vi "定时启动 (子VI).vi"   [LabVIEW 2016, in "斯坦道CODMn.lvlib"]
types:
  T1 = enum16{"启动测量", "标样核查", "零点核查", "跨度核查", "空白测试", "平行样测试", "加标回收", "空白校准", "标样校准", "初始化（清洗）", "停止测试", "仪器重启", "校时", "模式设置", "测量间隔设置"}
  T2 = cluster{"测量模式":enum16{"水样测量", "标样核查", "零点核查", "跨度核查", "空白测试", "加标回收", "平行样", "校零", "校标"}}
  T3 = cluster{"控制命令":enum16{"启动测量", "标样核查", "零点核查", "跨度核查", "空白测试", "平行样测试", "加标回收", "空白校准", "标样校准", "初始化（清洗）", "停止测试", "仪器重启", "校时", "模式设置", "测量间隔设置"}, "周期设置类型":enum16{"定点启动", "间隔启动"}, "定时功能启用":bool, "定时间隔":dbl, "24H周期设置":bool[], "零点核查时间":u16, "跨度核查时间":u16, "质控频次":enum16{"关闭", "每天", "星期一", "星期二", "星期三", "星期四", "星期五", "星期六", "星期日"}}
  T4 = enum16{"关闭", "每天", "星期一", "星期二", "星期三", "星期四", "星期五", "星期六", "星期日"}
  T5 = typedef "LVDateTimeRec.ctl" = cluster{"秒数的小数部分":dbl, "秒":i32, "分":i32, "时":i32, "日":i32, "月":i32, "年":i32, "天数（周）":i32, "天数（年）":i32, "DST":i32}
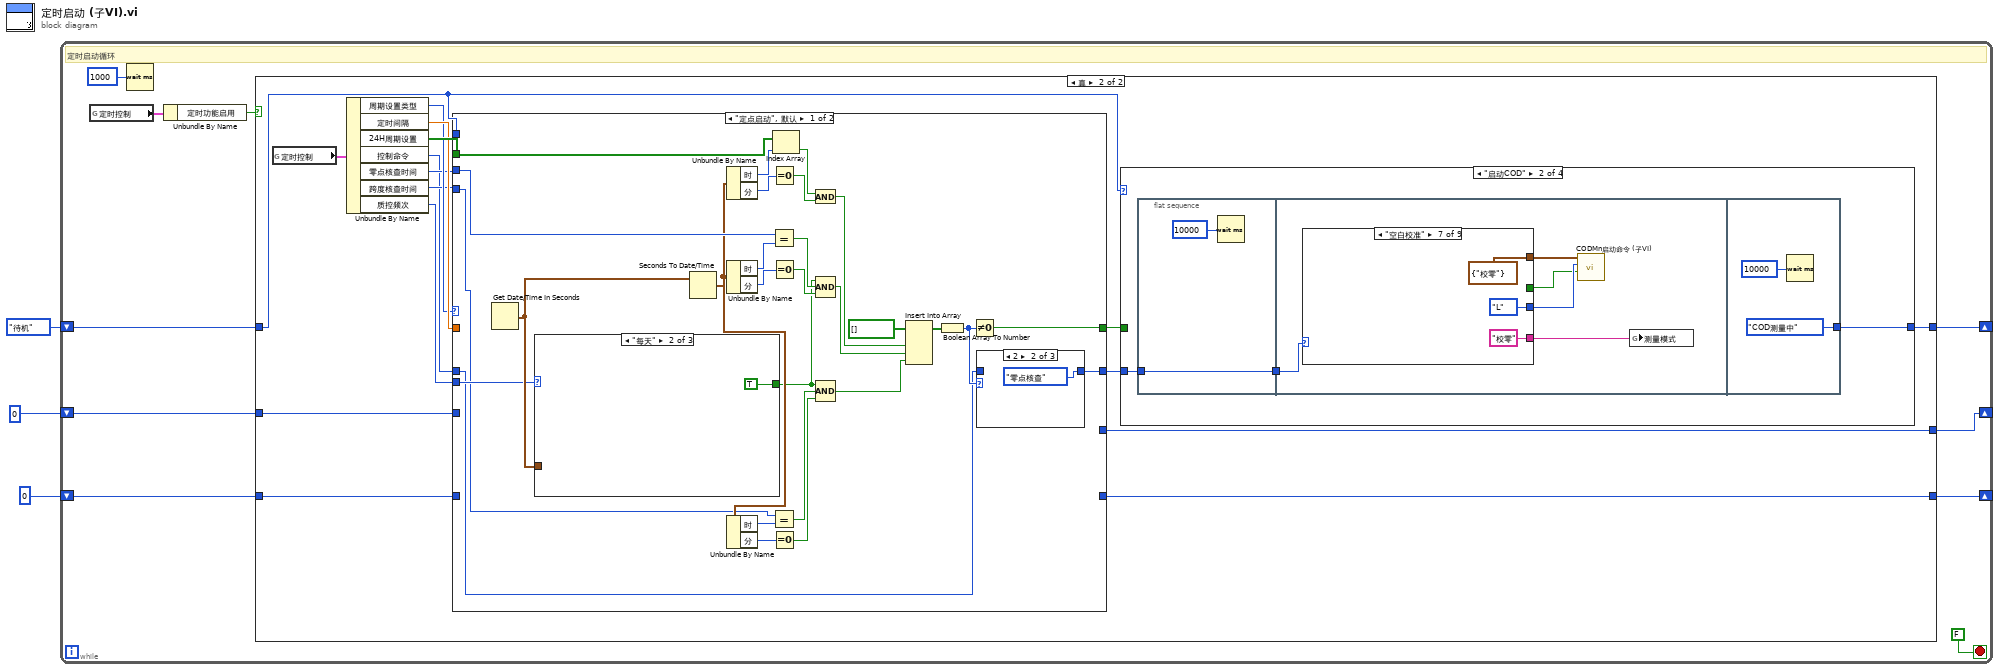
[diagram p0: block diagram]
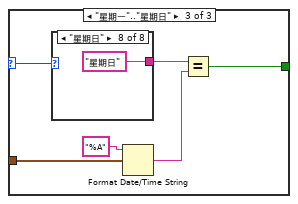
[diagram p4: hidden frame]
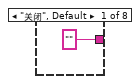
[diagram p5: hidden frame]
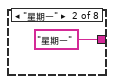
[diagram p6: hidden frame]
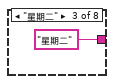
[diagram p7: hidden frame]
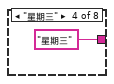
[diagram p8: hidden frame]
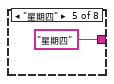
[diagram p9: hidden frame]
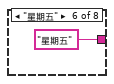
[diagram p10: hidden frame]
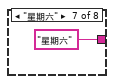
[diagram p11: hidden frame]
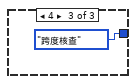
[diagram p13: hidden frame]
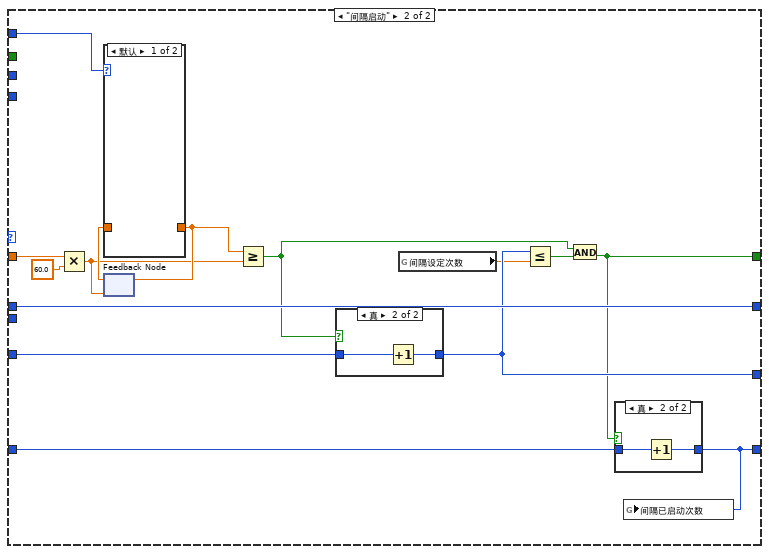
[diagram p14: hidden frame]
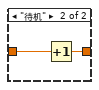
[diagram p17: hidden frame]
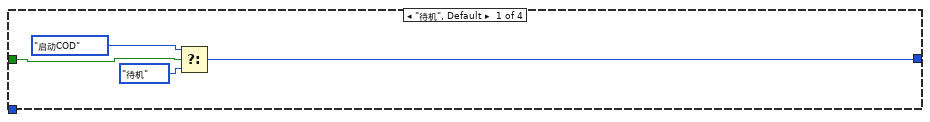
[diagram p18: hidden frame]
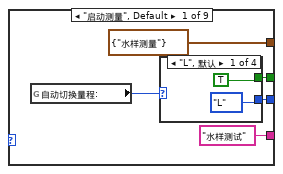
[diagram p19: hidden frame]
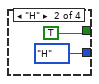
[diagram p20: hidden frame]
diagram:
  n1 = while {
    shift-right: [w12] -> _
    shift-left: enum16{"待机", "启动COD", "COD测量中", "延时"}."待机" -> [w11]
    shift-right: [w6] -> _
    shift-left: 0 -> [w7]
    shift-right: [w4] -> _
    shift-left: 0 -> [w5]
    stop <- FALSE stop-if-true
    # "定时启动循环"
    n2 = global read "CODMn断电保存全局变量.vi" "定时控制"() -> (w10:T3)
    n3 = Wait (ms)(milliseconds to wait=u32 1000 ("等待时间（毫秒）")) -> ()  [unwired: 1 out]
    n4 = Unbundle By Name(w10) -> ("定时功能启用"=w9:bool)
    n5 = case shown="真" w9 {
      tunnel: [w14 w30] -> w12
      tunnel: w11 -> [w14 w29]
      tunnel: w7 -> [_ w18]
      tunnel: [_ w17] -> w6
      tunnel: w5 -> [_ w16]
      tunnel: [_ w15] -> w4
      frame False {
      }
      frame True {
        n6 = global read "CODMn断电保存全局变量.vi" "定时控制"() -> (w23:T3)
        n7 = Unbundle By Name(w23) -> ("周期设置类型"=w24:enum16{"定点启动", "间隔启动"}, "定时间隔"=w25:dbl, "24H周期设置"=w26:bool[], "控制命令"=w19:T1, "零点核查时间"=w22:u16, "跨度核查时间"=w20:u16, "质控频次"=w21:T4)
        n8 = case shown="\"定点启动\", 默认" w24 {
          tunnel: w25 -> [_ w88]
          tunnel: w26 -> [w58 _]
          tunnel: w29 -> [_ w91]
          tunnel: [w34 w80] -> w28
          tunnel: w22 -> [w57 _]
          tunnel: w21 -> [w35 _]
          tunnel: w20 -> [w33 _]
          tunnel: w19 -> [w32 w85]
          tunnel: [w31 w85] -> w27
          tunnel: w18 -> [_ w84]
          tunnel: [_ w81] -> w17
          tunnel: w16 -> [_ w79]
          tunnel: [_ w77] -> w15
          frame "定点启动", Default {
            n9 = Get Date/Time In Seconds() -> (seconds since 1Jan1904=w53:timestamp)
            n10 = case shown="\"每天\"" w35 {
              selector: w35 -> [_ _ w63]
              tunnel: w53 -> [_ _ w64]
              tunnel: [_ TRUE w60] -> w42
              frame "关闭", Default {
              }
              frame "每天" {
              }
              frame "星期一".."星期日" {
                n11 = case shown="\"星期日\"" w63 {
                  tunnel: ["" ("时间格式字符串(%c)") "星期一" ("时间格式字符串(%c)") "星期二" ("时间格式字符串(%c)") "星期三" ("时间格式字符串(%c)") "星期四" ("时间格式字符串(%c)") "星期五" ("时间格式字符串(%c)") "星期六" ("时间格式字符串(%c)") "星期日" ("时间格式字符串(%c)")] -> w62
                  frame "关闭", Default {
                  }
                  frame "星期一" {
                  }
                  frame "星期二" {
                  }
                  frame "星期三" {
                  }
                  frame "星期四" {
                  }
                  frame "星期五" {
                  }
                  frame "星期六" {
                  }
                  frame "星期日" {
                  }
                }
                n12 = Format Date/Time String(time format string (%c)="%A" ("时间格式字符串(%c)"), seconds (now)=w64) -> (date/time string=w61:string)  [unwired: 1 in]
                n13 = Equal?(x=w62, y=w61) -> (x = y?=w60:bool)
              }
            }
            n14 = Seconds To Date/Time(time stamp (now)=w53) -> (date time rec=w43:T5)  [unwired: 1 in]
            n15 = Unbundle By Name(w43) -> ("时"=w56:i32, "分"=w55:i32)
            n16 = Unbundle By Name(w43) -> ("时"=w50:i32, "分"=w51:i32)
            n17 = Unbundle By Name(w43) -> ("时"=w45:i32, "分"=w44:i32)
            n18 = Equal?(x=w57, y=w50) -> (x = y?=w49:bool)
            n19 = Equal?(x=w33, y=w45) -> (x = y?=w46:bool)
            n20 = Equal To 0?(x=w55) -> (x = 0?=w54:bool)
            n21 = Equal To 0?(x=w51) -> (x = 0?=w48:bool)
            n22 = Equal To 0?(x=w44) -> (x = 0?=w47:bool)
            n23 = Index Array(array=w58, index=w56) -> (element=w52:bool)
            n24 = Compound Arithmetic op=AND ("复合运算")(w52, w54) -> (w40:bool)
            n25 = Compound Arithmetic op=AND ("复合运算")(w42, w49, w48) -> (w39:bool)
            n26 = Compound Arithmetic op=AND ("复合运算")(w42, w46, w47) -> (w38:bool)
            n27 = Insert Into Array(array=bool[] [], new element #1=w40, new element #2=w39, new element #3=w38) -> (w37:bool[])  [unwired: 1 in]
            n28 = Boolean Array To Number(Boolean array=w37) -> (number=w36:u32)
            n29 = Not Equal To 0?(x=w36) -> (x != 0?=w34:bool)
            n30 = case shown="2" w36 {
              tunnel: [w74 T1."零点核查" ("控制命令") T1."跨度核查" ("控制命令")] -> w31
              tunnel: w32 -> [w74 _ _]
              frame 0, Default {
              }
              frame 2 {
              }
              frame 4 {
              }
            }
          }
          frame "间隔启动" {
            n31 = Multiply(x=w88, y=60.0) -> (x*y=w86:dbl)
            n32 = feedback #1(w86) -> (w90:dbl)
            n33 = case shown="默认" w91 {
              tunnel: w90 -> [_ w99]
              tunnel: [_ w98] -> w89
              frame Default {
              }
              frame "待机" {
                n34 = Increment(x=w99) -> (x+1=w98:dbl)
              }
            }
            n35 = feedback-in #1(w89) -> ()
            n36 = Greater Or Equal?(x=w89, y=w86) -> (x >= y?=w82:bool)
            n37 = case shown="真" w82 {
              tunnel: w84 -> [w95 w97]
              tunnel: [w95 w96] -> w81
              frame False {
              }
              frame True {
                n38 = Increment(x=w97) -> (x+1=w96:i32)
              }
            }
            n39 = global read "CODMn断电保存全局变量.vi" "间隔设定次数"() -> (w78:dbl)
            n40 = Less Or Equal?(x=w81, y=w78) -> (x <= y?=w83:bool)
            n41 = And(x=w82, y=w83) -> (x .and. y?=w80:bool)
            n42 = case shown="真" w80 {
              tunnel: w79 -> [w92 w94]
              tunnel: [w92 w93] -> w77
              frame False {
              }
              frame True {
                n43 = Increment(x=w94) -> (x+1=w93:i32)
              }
            }
            n44 = global write "CODMn断电保存全局变量.vi" "间隔已启动次数"(w77) -> ()
          }
        }
        n45 = case shown="\"启动COD\"" w29 {
          tunnel: [w100 w106 w158 enum16{"待机", "启动COD", "COD测量中", "延时"}."待机"] -> w30
          tunnel: w28 -> [w103 _ _ _]
          tunnel: w27 -> [_ w104 _ _]
          frame "待机", Default {
            n46 = Select(t=enum16{"待机", "启动COD", "COD测量中", "延时"}."启动COD", s=w103, f=enum16{"待机", "启动COD", "COD测量中", "延时"}."待机") -> (s? t:f=w100:enum16{"待机", "启动COD", "COD测量中", "延时"})
          }
          frame "启动COD" {
            n47 = flat-sequence {
              tunnel: w104 -> [w108]
              tunnel: [w108] -> w105
              tunnel: w105 -> [w113]
              tunnel: [enum16{"待机", "启动COD", "COD测量中", "延时"}."COD测量中"] -> w106
              frame #0 {
                n48 = Wait (ms)(milliseconds to wait=u32 10000 ("等待时间（毫秒）")) -> ()  [unwired: 1 out]
              }
              frame #1 {
                n49 = case shown="\"空白校准\"" w113 {
                  tunnel: [T2 {"测量模式"=enum."水样测量"} ("启动测量模式") T2 {"测量模式"=enum."标样核查"} ("启动测量模式") T2 {"测量模式"=enum."空白测试"} ("启动测量模式") T2 {"测量模式"=enum."跨度核查"} ("启动测量模式") T2 {"测量模式"=enum."加标回收"} ("启动测量模式") T2 {"测量模式"=enum."平行样"} ("启动测量模式") T2 {"测量模式"=enum."校零"} ("启动测量模式") T2 {"测量模式"=enum."校标"} ("启动测量模式") T2 {"测量模式"=enum."零点核查"} ("启动测量模式")] -> w112
                  tunnel: ["水样测试" ("测量模式") "标样核查" ("测量模式") "空白测试" ("测量模式") "跨度核查" ("测量模式") "加标回收" ("测量模式") "平行样" ("测量模式") "校零" ("测量模式") "校标" ("测量模式") "零点核查" ("测量模式")] -> w111
                  tunnel: [w116 w127 enum32{"H", "L", "AUTO"}."L" ("CODMn跨度量程选择") w133 enum32{"H", "L", "AUTO"}."AUTO" ("CODMn跨度量程选择") enum32{"H", "L", "AUTO"}."AUTO" ("CODMn跨度量程选择") enum32{"H", "L", "AUTO"}."L" ("CODMn跨度量程选择") enum32{"H", "L", "AUTO"}."AUTO" ("CODMn跨度量程选择") w148] -> w110
                  tunnel: [w115 _ _ _ _ _ _ _ _] -> w109
                  frame "启动测量", Default {
                    n50 = global read "CODMn断电保存全局变量.vi" "自动切换量程:"() -> (w114:enum16{"L", "H", "自动切换测一次", "自动切换测两次"})
                    n51 = case shown="\"L\", 默认" w114 {
                      tunnel: [enum32{"H", "L", "AUTO"}."L" ("CODMn跨度量程选择") enum32{"H", "L", "AUTO"}."H" ("CODMn跨度量程选择") enum32{"H", "L", "AUTO"}."AUTO" ("CODMn跨度量程选择") enum32{"H", "L", "AUTO"}."AUTO" ("CODMn跨度量程选择")] -> w116
                      tunnel: [TRUE TRUE FALSE FALSE] -> w115
                      frame "L", Default {
                      }
                      frame "H" {
                      }
                      frame "自动切换测一次" {
                      }
                      frame "自动切换测两次" {
                      }
                    }
                  }
                  frame "标样核查" {
                    n52 = global read "CODMn断电保存全局变量.vi" "标样核查量程选择"() -> (w127:enum32{"H", "L", "AUTO"})
                  }
                  frame "空白测试" {
                  }
                  frame "跨度核查" {
                    n53 = global read "CODMn断电保存全局变量.vi" "CODMn跨度量程选择"() -> (w133:enum32{"H", "L", "AUTO"})
                  }
                  frame "加标回收" {
                  }
                  frame "平行样测试" {
                  }
                  frame "空白校准" {
                  }
                  frame "标样校准" {
                  }
                  frame "零点核查" {
                    n54 = global read "CODMn断电保存全局变量.vi" "零点核查量程选择"() -> (w148:enum32{"H", "L", "AUTO"})
                  }
                }
                n55 = call "CODMn启动命令 (子VI).vi"("强制切换"=w109, "CODMn量程切换"=w110, "启动测量模式"=w112) -> ()  [unwired: 9 in]
                n56 = global write "COD测量模式全局.vi" "测量模式"(w111) -> ()
              }
              frame #2 {
                n57 = Wait (ms)(milliseconds to wait=u32 10000 ("等待时间（毫秒）")) -> ()  [unwired: 1 out]
              }
            }
          }
          frame "COD测量中" {
            n58 = global read "运行时序全局变量.vi" "多列列表框"() -> (w157:i32)
            n59 = Equal?(x=w157, y=0) -> (x = y?=w155:bool)
            n60 = Select(t=enum16{"待机", "启动COD", "COD测量中", "延时"}."延时", s=w155, f=enum16{"待机", "启动COD", "COD测量中", "延时"}."COD测量中") -> (s? t:f=w158:enum16{"待机", "启动COD", "COD测量中", "延时"})
          }
          frame "延时" {
            n61 = Wait (ms)(milliseconds to wait=u32 5000 ("等待时间（毫秒）")) -> ()  [unwired: 1 out]
          }
        }
      }
    }
  }
